vi "Destroy Observer.vi"(11 "observer in":T1) -> ()   [LabVIEW 2014, in "Observable Actor.lvlib" / "Observable Actor.lvclass"]
uses:
  Observable Actor.lvclass
  Observer.ctl
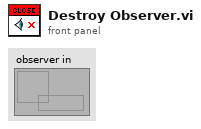
[diagram p1: front panel]
types:
  T1 = typedef "Observable Actor.lvlib/Observable Actor.lvclass/Observer.ctl" = refnum<queue>
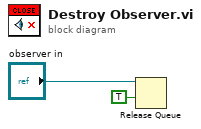
[diagram p0: block diagram]
diagram:
  n1 = Release Queue(queue="observer in", force destroy? (F)=TRUE) -> ()  [unwired: 1 in, 3 out]
